vi "Setup servo out.vi"(7 "buffer size multiple":dbl=2.0, 8 "error in (no error)":errorcluster, 10 "Run info in":T1, 11 "Sampling info in":T2={"Channels"=[], "Sampling freq"=0, "Output freq"=0, "Update freq"=0, "Steps per rev"=0, "Counts per rev"=0, "Amplifier"="", "Motor driver"="", "Step bit"=0, "Max speed"=0.0, "Max accel"=0.0, "Pos gain"=0.0, "Vel gain"=0.0, "counter"="Dev1/ctr0"} {"Channels"."Hi cutoff" items=["500"=500.0, "1k"=1000.0, "5k"=5000.0, "10k"=10000.0, "20k"=20000.0]; "Channels"."Lo cutoff" items=["0.1"=0.1, "1"=1.0, "10"=10.0, "100"=100.0, "300"=300.0]; "Channels"."Gain" items=["x100"=100, "x1000"=1000, "x10000"=10000]}) -> (0 "error out":errorcluster, 1 "output delay":dbl, 2 "Run info":T1, 3 "Sampling info out":T2={"Channels"=[], "Sampling freq"=0, "Output freq"=0, "Update freq"=0, "Steps per rev"=0, "Counts per rev"=0, "Amplifier"="", "Motor driver"="", "Step bit"=0, "Max speed"=0.0, "Max accel"=0.0, "Pos gain"=0.0, "Vel gain"=0.0, "counter"="Dev1/ctr0"} {"Channels"."Hi cutoff" items=["500"=500.0, "1k"=1000.0, "5k"=5000.0, "10k"=10000.0, "20k"=20000.0]; "Channels"."Lo cutoff" items=["0.1"=0.1, "1"=1.0, "10"=10.0, "100"=100.0, "300"=300.0]; "Channels"."Gain" items=["x100"=100, "x1000"=1000, "x10000"=10000]})   [LabVIEW 2012]
uses:
  Sampling info.ctl
  Channel.ctl
  Run info.ctl
  <vilib>/DAQmx/write.llb/DAQmx Write (Counter 1D Frequency 1Chan NSamp).vi
  <vilib>/DAQmx/create/channels.llb/DAQmx Create Channel (CO-Pulse Generation-Frequency).vi
  <vilib>/DAQmx/configure/timing.llb/DAQmx Timing (Implicit).vi
  <vilib>/DAQmx/miscellaneous.llb/DAQmx Fill In Error Info.vi
  <resource>/objmgr/daqmx.rc
panel:
  out "number of samples written per channel":u32
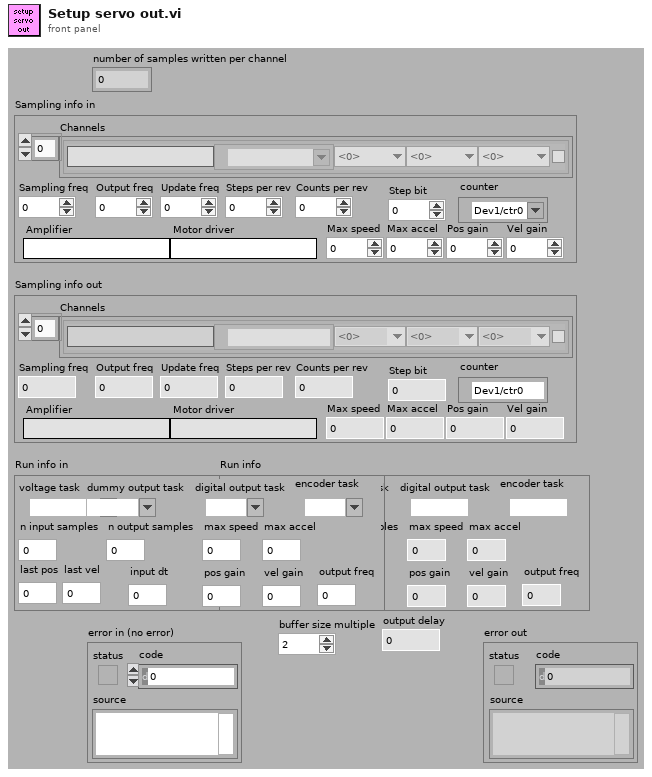
[diagram p1: front panel]
types:
  T1 = typedef "Run info.ctl" = cluster{"voltage task":refnum<k21>, "dummy output task":refnum<k21>, "digital output task":refnum<k21>, "encoder task":refnum<k21>, "n input samples":i32, "n output samples":i32, "max speed":dbl, "max accel":dbl, "last pos":dbl, "last vel":dbl, "pos gain":dbl, "vel gain":dbl, "input dt":dbl, "output freq":dbl}
  T2 = typedef "Sampling info.ctl" = cluster{"Channels":T3[], "Sampling freq":i32, "Output freq":i32, "Update freq":i32, "Steps per rev":i32, "Counts per rev":i32, "Amplifier":string, "Motor driver":string, "Step bit":u8, "Max speed":dbl, "Max accel":dbl, "Pos gain":dbl, "Vel gain":dbl, "counter":tag}
  T3 = typedef "Channel.ctl" = cluster{"Name":string, "Chan":tag, "Gain":u16, "Lo cutoff":dbl, "Hi cutoff":dbl, "Notch":bool}
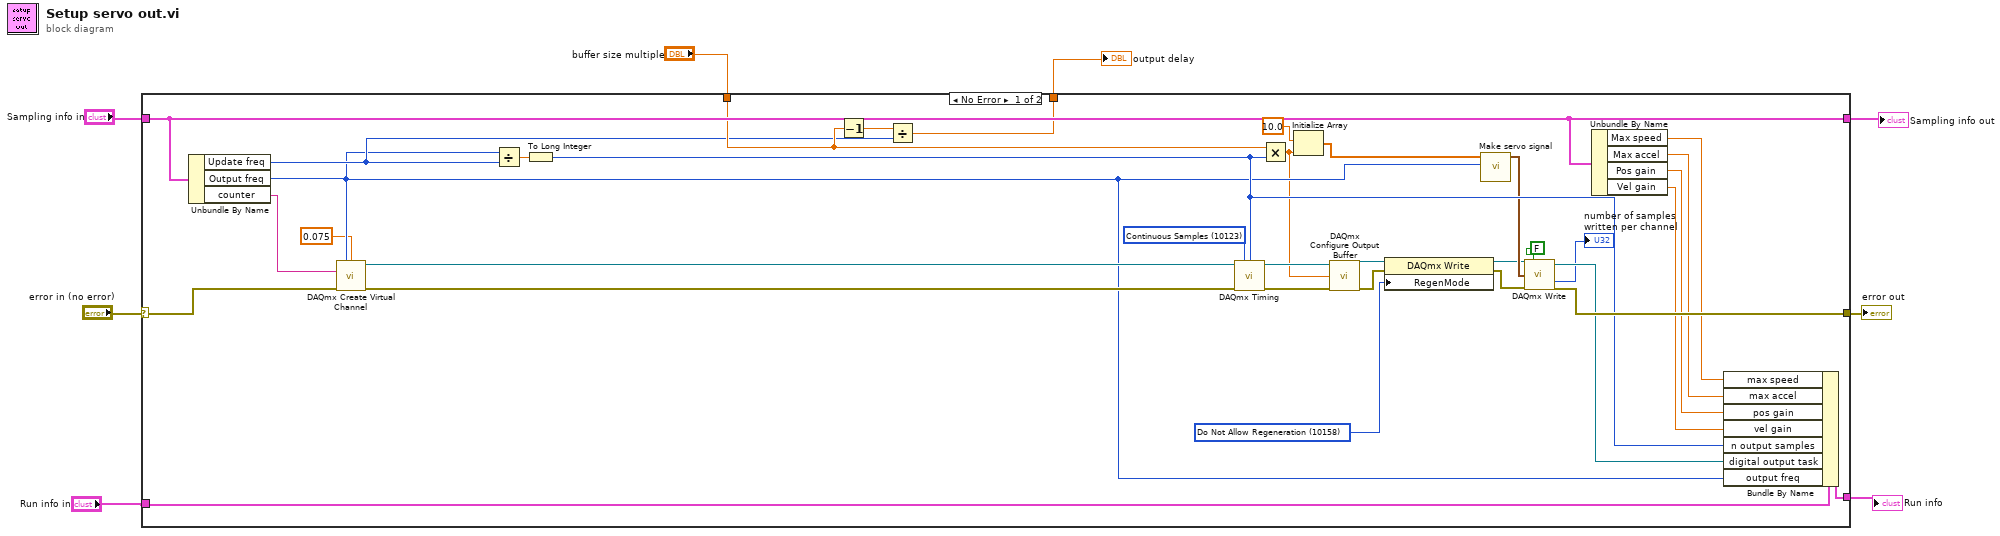
[diagram p0: block diagram]
diagram:
  n1 = case shown="No Error" "error in (no error)" {
    selector: "error in (no error)" -> [w26 w45]
    tunnel: [w43 w44] -> w4
    tunnel: [w38 w45] -> w7
    tunnel: [w35 w46] -> w3
    tunnel: "Sampling info in" -> [w35 w46]
    tunnel: "Run info in" -> [w42 w44]
    tunnel: "buffer size multiple" -> [w30 _]
    tunnel: [w29 _] -> w1
    frame No Error {
      w11 = 10158 items=["Allow Regeneration"=10097, "Do Not Allow Regeneration"=10158] ("RegenMode")
      w19 = 10123 items=["Finite Samples"=10178, "Continuous Samples"=10123, "Hardware Timed Single Point"=12522] ("sample mode")
      n2 = Unbundle By Name(w35) -> ("Update freq"=w23:i32, "Output freq"=w21:i32, "counter"=w20:tag)
      n3 = call-poly <vilib>:"DAQmx Create Virtual Channel.vi"("frequency"=w21, "duty cycle"=0.075, "counter"=w20, "error in"=w26) -> ("task out"=w27:refnum<k21>, "error out"=w25:errorcluster)  [unwired: 10 in]
      n4 = Divide(x=w21, y=w23) -> (x/y=w41:dbl)
      n5 = To Long Integer(number=w41) -> (32bit integer=w36:i32)
      n6 = Decrement(x=w30) -> (x-1=w28:dbl)
      n7 = Divide(x=w28, y=w23) -> (x/y=w29:dbl)
      n8 = call-poly <vilib>:"DAQmx Timing.vi"("task/channels in"=w27, "sample mode"=w19, "samples per channel"=w36, "error in"=w25) -> ("task out"=w17:refnum<k21>, "error out"=w15:errorcluster)  [unwired: 10 in]
      n9 = Multiply(x=w30, y=w36) -> (x*y=w16:dbl)
      n10 = Initialize Array(10.0 ("element"), w16) -> (w24:dbl[])
      n11 = call <vilib>:"DAQmx Configure Output Buffer.vi"("task/channels in"=w17, "buffer size (in samples per channel)"=w16, "error in"=w15) -> ("task out"=w13:refnum<k21>, "error out"=w12:errorcluster)  [unwired: 11 in]
      n12 = property class="DAQmx Write"(reference=w13, error in=w12, "RegenMode"=w11) -> (reference out=w10:refnum<k21>, error out=w9:errorcluster)
      n13 = call "Make servo signal.vi"("sampling frequency"=w21, "Data"=w24) -> ("sine PWM pattern"=w22:cluster{"duty cycle":dbl, "frequency":dbl}[])  [unwired: 7 in, 2 out]
      n14 = call-poly <vilib>:"DAQmx Write.vi"("task/channels in"=w10, "auto start"=FALSE, "data"=w22, "error in"=w9) -> ("task out"=w37:refnum<k21>, "number of samples written per channel"=→"number of samples written per channel":u32, "error out"=w38:errorcluster)  [unwired: 9 in]
      n15 = Unbundle By Name(w35) -> ("Max speed"=w34:dbl, "Max accel"=w33:dbl, "Pos gain"=w32:dbl, "Vel gain"=w31:dbl)
      n16 = Bundle By Name(cluster=w42, "max speed"=w34, "max accel"=w33, "pos gain"=w32, "vel gain"=w31, "n output samples"=w36, "digital output task"=w37, "output freq"=w21) -> (w43:T1)
    }
    frame Error {
    }
  }
  "error out" <- w7
  "Run info" <- w4
  "Sampling info out" <- w3
  "output delay" <- w1
